vi "CD Init_Get Status Channels Reference.vi"(8 "error in (no error)":errorcluster, 11 "Device Reference":T2 format="%.0x") -> (0 "error out":errorcluster, 3 "Array":T1[](array[typedef]) format="%.0x")   [LabVIEW 2020, in "Ballard MIL-1553 Engine.lvlib"]
doc: "This VI gets references for all Status Channels used."
uses:
  Ballard MIL-1553 Engine.lvlib
  <vilib>/NI VeriStand/Custom Device API/Custom Device Item Ref.ctl
  <vilib>/NI VeriStand/Custom Device API/Data Reference.ctl
  <vilib>/NI VeriStand/Custom Device API/Data Access Type.ctl
  Shared/Controls and Global/Global.vi
  <vilib>/NI VeriStand/Custom Device Tools/Custom Device Utility Library/NI VeriStand - Search for Item by GUID.vi
  <vilib>/NI VeriStand/Custom Device API/Custom Device API.lvlib
  <vilib>/NI VeriStand/Custom Device Tools/Custom Device Utility Library/Custom Device Utility Library.lvlib
  Shared/Ballard 1553 Shared.lvlib
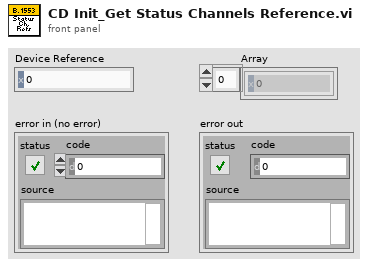
[diagram p1: front panel]
types:
  T1 = typedef "Custom Device API.lvlib/Data Reference.ctl" = i32
  T2 = typedef "Custom Device API.lvlib/Custom Device Item Ref.ctl" = u64
  T3 = typedef "Custom Device API.lvlib/Data Access Type.ctl" = enum16{"Read", "Write"}
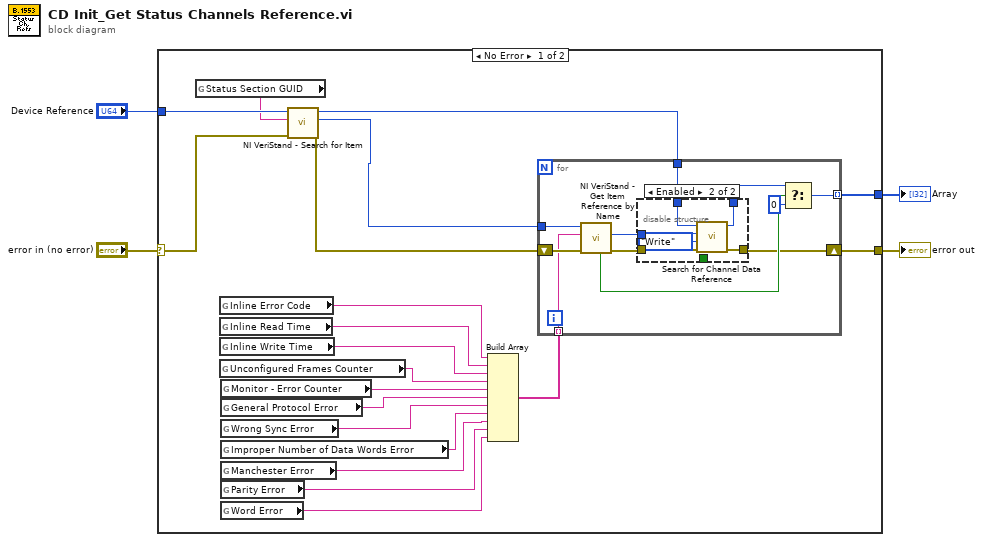
[diagram p0: block diagram]
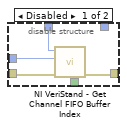
[diagram p2: hidden frame]
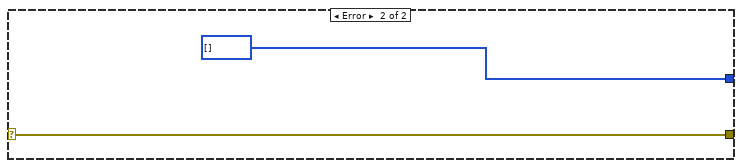
[diagram p3: hidden frame]
diagram:
  n1 = case shown="No Error" "error in (no error)" {
    selector: "error in (no error)" -> [w22 w48]
    tunnel: [w11 w48] -> w4
    tunnel: "Device Reference" -> [w23 _]
    tunnel: [w5 T1[] []] -> w2
    frame No Error {
      n2 = global read "Global.vi" "Status Section GUID"() -> (w21:string)
      n3 = global read "Global.vi" "Inline Error Code"() -> (w10:string)
      n4 = global read "Global.vi" "Inline Read Time"() -> (w9:string)
      n5 = global read "Global.vi" "Inline Write Time"() -> (w8:string)
      n6 = global read "Global.vi" "Unconfigured Frames Counter"() -> (w7:string)
      n7 = global read "Global.vi" "Monitor - Error Counter"() -> (w12:string)
      n8 = global read "Global.vi" "General Protocol Error"() -> (w13:string)
      n9 = global read "Global.vi" "Wrong Sync Error"() -> (w14:string)
      n10 = global read "Global.vi" "Improper Number of Data Words Error"() -> (w15:string)
      n11 = global read "Global.vi" "Manchester Error"() -> (w16:string)
      n12 = global read "Global.vi" "Parity Error"() -> (w17:string)
      n13 = global read "Global.vi" "Word Error"() -> (w18:string)
      n14 = call-poly <vilib>:"NI VeriStand - Search for Item.vi"("error in"=w22, "Item GUID"=w21, "Section Ref in"=w23) -> ("error out"=w24:errorcluster, "Item Ref"=w20:T2, "Section Ref out"=w19:T2)  [unwired: 5 in, 1 out]
      n15 = Build Array(w10, w9, w8, w7, w12, w13, w14, w15, w16, w17, w18) -> (w6:string[])
      n16 = for {
        tunnel: w20 -> [w29]
        tunnel: w19 -> [w28]
        tunnel: w6 -> [w26] mode=indexing
        shift-right: [w27] -> w11
        shift-left: w24 -> [w34]
        tunnel: [w25] -> w5 mode=indexing
        n17 = call <vilib>:"NI VeriStand - Get Item Reference by Name.vi"("error in (no error)"=w34, "Item Name"=w26, "Parent Ref in"=w29) -> ("error out"=w30:errorcluster, "Item Ref"=w31:T2, "Found"=w33:bool)  [unwired: 5 in, 1 out]
        n18 = disable-structure shown="Enabled" {
          disable-tunnel: w30 -> [w40 w46]
          disable-tunnel: [w39 _] -> _
          disable-tunnel: [w38 w43] -> w27
          disable-tunnel: w28 -> [w37 w45]
          disable-tunnel: w31 -> [w36 w44]
          disable-tunnel: [_ w42] -> w32
          frame Disabled {
            n19 = call <vilib>:"NI VeriStand - Get Channel FIFO Buffer Index.vi"("error in"=w40, "Channel Ref"=w36, "Device Ref in"=w37) -> ("error out"=w38:errorcluster, "Found"=w39:bool)  [unwired: 4 in, 3 out]
          }
          frame Enabled {
            n20 = call "Search for Channel Data Reference.vi"("error in (no error)"=w46, "Access"=Data_Access_Type."Write", "Item Ref"=w44, "Device Ref in"=w45) -> ("error out"=w43:errorcluster, "Channel Data Reference"=w42:T1)  [unwired: 6 in]
          }
        }
        n21 = Select(t=w32, s=w33, f=T1 0) -> (s? t:f=w25:T1)
      }
    }
    frame Error {
    }
  }
  "error out" <- w4
  "Array" <- w2
